vi "Forward_Kinematics (geo and matrix).vi"(8 "geometry":cluster{"L 1":dbl, "L 2":dbl, "q":dbl[]}={"L 1"=30.0, "L 2"=35.0, "q"=[20.0, -40.0]}, 9 "geometry?":bool, 10 "arms":T1(array[cluster])=[{"Translation"={"X"=0.0, "Y"=0.0, "Z"=0.0}, "Axis"=enum."z", "Angle (degrees)"=20.0}, {"Translation"={"X"=30.0, "Y"=0.0, "Z"=0.0}, "Axis"=enum."z", "Angle (degrees)"=-40.0}, {"Translation"={"X"=35.0, "Y"=0.0, "Z"=0.0}, "Axis"=enum."z", "Angle (degrees)"=0.0}] {"Angle (degrees)" scale=0.0..180.0}, 11 "picture in":picture) -> (0 "end (2D)":cluster{"x":dbl, "y":dbl}, 1 "end effector":cluster{"X":dbl, "Y":dbl}={"X"=61.080020351084045, "Y"=-1.710100716628343}, 3 "2D Picture":picture)   [LabVIEW 2024]
uses:
  <vilib>/Analysis/Matrix/Datatypes/RealMatrix.ctl
  <vilib>/Analysis/baseanly.llb/Real A x B.vi
  <vilib>/Analysis/NI_AALBase.lvlib
  <vilib>/Analysis/Matrix/NI_Matrix.lvlib
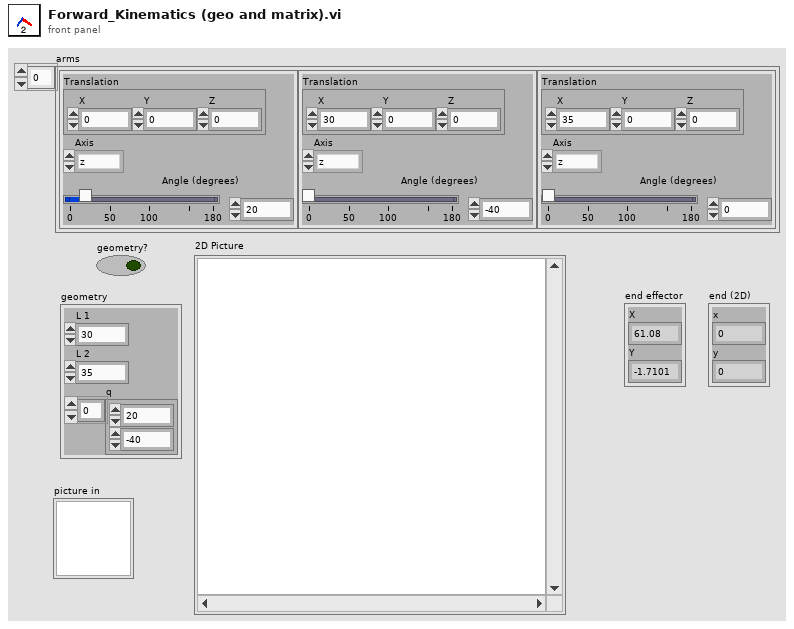
[diagram p1: front panel]
types:
  T1 = cluster{"Translation":cluster{"X":dbl, "Y":dbl, "Z":dbl}, "Axis":enum16{"x", "y", "z"}, "Angle (degrees)":dbl}[]
  T2 = typedef "NI_Matrix.lvlib/RealMatrix.ctl" = dbl[][]
  T3 = cluster{"Real Matrix Element":dbl, "Real Matrix Element":dbl}
  T4 = cluster{"Real Matrix Element":dbl, "Real Matrix Element":dbl}[]
  T5 = cluster{"Width":u16, "Style":enum32{"Solid", "Dash", "Dot", "DashDot", "DashDotDot"}}
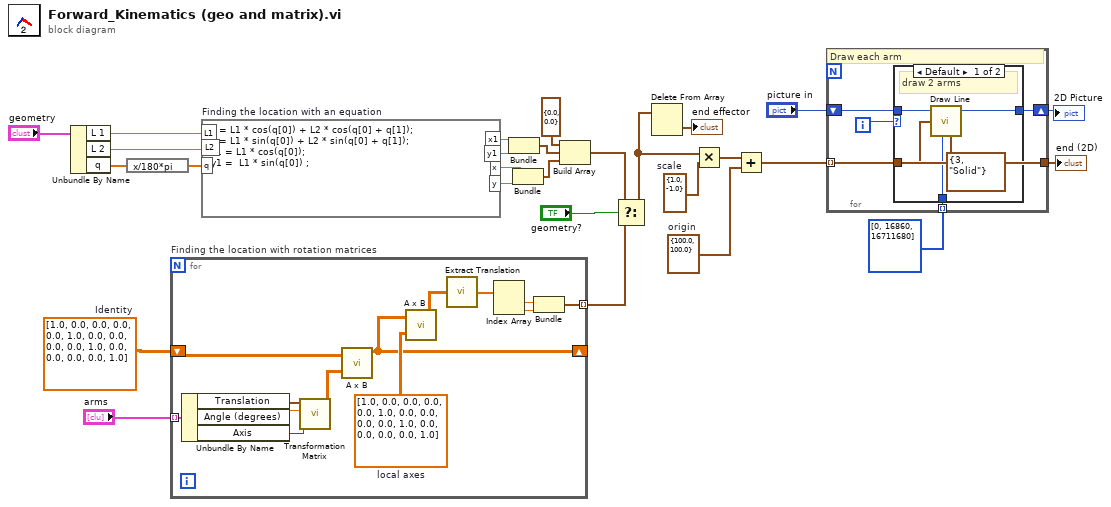
[diagram p0: block diagram]
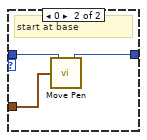
[diagram p2: hidden frame]
diagram:
  w8 = T2 [[1.0, 0.0, 0.0, 0.0], [0.0, 1.0, 0.0, 0.0], [0.0, 0.0, 1.0, 0.0], [0.0, 0.0, 0.0, 1.0]]  # Identity
  w13 = cluster{"x":dbl, "y":dbl} {"x"=1.0, "y"=-1.0}  # scale
  w12 = cluster{"x":dbl, "y":dbl} {"x"=100.0, "y"=100.0}  # origin
  n1 = Unbundle By Name("geometry") -> ("L 1"=w24:dbl, "L 2"=w25:dbl, "q"=w26:dbl[])
  n2 = expression code="x/180*pi"(w26) -> (w4:dbl[])
  n3 = for "Finding the location with rotation matrices" {
    tunnel: "arms" -> [w35] mode=indexing
    shift-right: [w33] -> _
    shift-left: w8 -> [w34]
    tunnel: [w28] -> w7 mode=indexing
    w36 = T2 [[1.0, 0.0, 0.0, 0.0], [0.0, 1.0, 0.0, 0.0], [0.0, 0.0, 1.0, 0.0], [0.0, 0.0, 0.0, 1.0]]  # local axes
    n4 = Unbundle By Name(w35) -> ("Translation"=w40:cluster{"X":dbl, "Y":dbl, "Z":dbl}, "Angle (degrees)"=w39:dbl, "Axis"=w38:enum16{"x", "y", "z"})
    n5 = call <userlib>:"Transformation Matrix.vi"("Axis"=w38, "Angle (degrees)"=w39, "Translation"=w40) -> ("Transformation Matrix"=w37:T2)  [unwired: 8 in]
    n6 = call-poly <vilib>:"A x B.vi"("B"=w37, "A"=w34) -> ("A x B"=w33:T2)  [unwired: 1 out]
    n7 = call-poly <vilib>:"A x B.vi"("B"=w36, "A"=w33) -> ("A x B"=w32:T2)  [unwired: 1 out]
    n8 = call <userlib>:"Extract Translation.vi"("Transformation matrix"=w32) -> ("translation"=w31:dbl[])
    n9 = Index Array(array=w31) -> (element #1=w30:dbl, element #2=w29:dbl)  [unwired: 2 in]
    n10 = Bundle("Real Matrix Element"=w30, "Real Matrix Element"=w29) -> (w28:T3)  [unwired: 1 in]
  }
  n11 = formula code="x = L1 * cos(q[0]) + L2 * cos(q[0] + q[1]);\ny = L1 * sin(q[0]) + L2 * sin(q[0] + q[1]);\nx1 = L1 * cos(q[0]);\ny1 =  L1 * sin(q[0]) ;" "Finding the location with an equation"("q"=w4, "L1"=w24, "L2"=w25) -> ("x"=w23:dbl, "y"=w22:dbl, "x1"=w21:dbl, "y1"=w20:dbl)
  n12 = Bundle("x1"=w21, "y1"=w20) -> (w19:cluster{"x1":dbl, "y1":dbl})  [unwired: 1 in]
  n13 = Bundle("x"=w23, "y"=w22) -> (w18:cluster{"x":dbl, "y":dbl})  [unwired: 1 in]
  n14 = Build Array(cluster{"x":dbl, "y":dbl} {"x"=0.0, "y"=0.0} ("y"), w19, w18) -> (w6:cluster{"x":dbl, "y":dbl}[])
  n15 = Select(t=w6, s="geometry?", f=w7) -> (s? t:f=w3:T4)
  n16 = Delete From Array(array=w3) -> (deleted portion=→"end effector":T3)  [unwired: 2 in, 1 out]
  n17 = Multiply(x=w3, y=w13) -> (x*y=w11:cluster{dbl, dbl}[])
  n18 = Add(x=w11, y=w12) -> (x+y=w10:cluster{dbl, dbl}[])
  n19 = for {
    shift-right: [w43] -> w16
    shift-left: "picture in" -> [w44]
    tunnel: u32[] [0, 16860, 16711680] -> [w42] mode=indexing
    tunnel: w10 -> [w41] mode=indexing
    tunnel: [w41] -> w1
    i -> [w45]
    # "Draw each arm"
    n20 = case shown="Default" w45 {
      tunnel: w44 -> [w50 w53]
      tunnel: [w49 w52] -> w43
      tunnel: w41 -> [w48 w51]
      tunnel: w42 -> [w47 _]
      frame Default {
        # "draw 2 arms"
        n21 = call <vilib>:"Draw Line.vi"("picture"=w50, "end point"=w48, "color(black)"=w47, "pen"=T5 {"Width"=3, "Style"=enum."Solid"}) -> ("new picture"=w49:picture)  [unwired: 5 in]
      }
      frame 0 {
        # "start at base"
        n22 = call <vilib>:"Move Pen.vi"("new position"=w51, "picture"=w53) -> ("new picture"=w52:picture)  [unwired: 3 in]
      }
    }
  }
  "2D Picture" <- w16
  "end (2D)" <- w1
